vi "fgv_pc_lidar_data.vi"(7 "cmd":enum16{"init", "read", "write"}(ring), 11 "Lidar array in":cluster{"x":dbl, "y":dbl}[](array[cluster])) -> (3 "Lidar array out":cluster{"x":dbl, "y":dbl}[](array[cluster]))   [LabVIEW 2019]
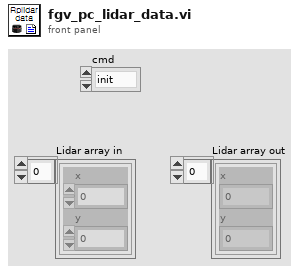
[diagram p1: front panel]
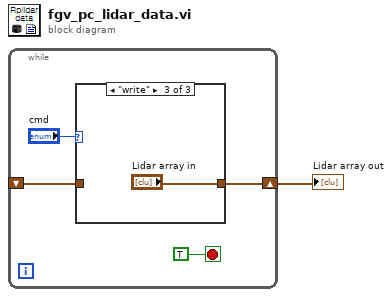
[diagram p0: block diagram]
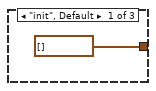
[diagram p2: hidden frame]
diagram:
  n1 = while {
    shift-right: [w3] -> w1
    shift-left: _ -> [w2]
    stop <- TRUE stop-if-true
    n2 = case shown="\"write\"" "cmd" {
      tunnel: [cluster{"x":dbl, "y":dbl}[] [] ("appended array") w7 "Lidar array in"] -> w3
      tunnel: w2 -> [_ w7 _]
      frame "init", Default {
      }
      frame "read" {
      }
      frame "write" {
      }
    }
  }
  "Lidar array out" <- w1
